vi "18-2.vi"() -> ()   [LabVIEW 2019, in "18.lvlib"]
uses:
  18.lvlib
panel:
  out "Snailfish Number x+y":string
  out "Snailfish Number y":string
  in  "Sample?":bool
  out "Max Snailfish Number Sum Magnitude":u64
  in  "Sample Index":i32
  out "Snailfish Number x":string
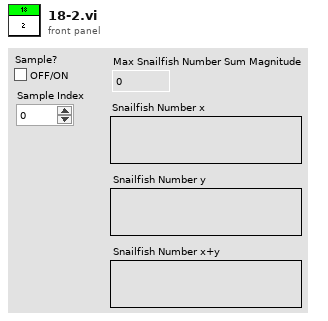
[diagram p1: front panel]
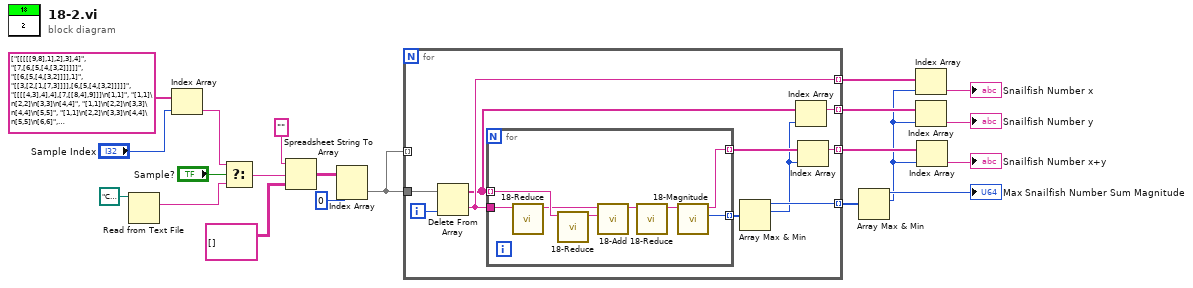
[diagram p0: block diagram]
diagram:
  n1 = Read from Text File(file (use dialog)=path "C:/Users/craig.walker/Documents/GitHub/lv2019-Advent-of-Code-2021/18/input.txt") -> (text=w12:string)  [unwired: 3 in, 3 out]
  n2 = Index Array(array=string[] ["[[[[[9,8],1],2],3],4]", "[7,[6,[5,[4,[3,2]]]]]", "[[6,[5,[4,[3,2]]]],1]", "[[3,[2,[1,[7,3]]]],[6,[5,[4,[3,2]]]]]", "[[[[4,3],4],4],[7,[[8,4],9]]]\n[1,1]", "[1,1]\n[2,2]\n[3,3]\n[4,4]", "[1,1]\n[2,2]\n[3,3]\n[4,4]\n[5,5]", "[1,1]\n[2,2]\n[3,3]\n[4,4]\n[5,5]\n[6,6]", "[[[0,[4,5]],[0,0]],[[[4,5],[2,6]],[9,5]]]\n[7,[[[3,7],[4,3]],[[6,3],[8,8]]]]\n[[2,[[0,8],[3,4]]],[[[6,7],1],[7,[1,6]]]]\n[[[[2,4],7],[6,[0,5]]],[[[6,8],[2,8]],[[2,1],[4,5]]]]\n[7,[5,[[3,8],[1,4]]]]\n[[2,[2,2]],[8,[8,1]]]\n[2,9]\n[1,[[[9,3],9],[[9,0],[0,7]]]]\n[[[5,[7,4]],7],1]\n[[[[4,2],2],6],[8,7]]", "[9,1]", "[[[0,[5,8]],[[1,7],[9,6]]],[[4,[1,2]],[[1,4],2]]]\n[[[5,[2,8]],4],[5,[[9,9],0]]]\n[6,[[[6,2],[5,6]],[[7,6],[4,7]]]]\n[[[6,[0,7]],[0,9]],[4,[9,[9,0]]]]\n[[[7,[6,4]],[3,[1,3]]],[[[5,5],1],9]]\n[[6,[[7,3],[3,2]]],[[[3,8],[5,7]],4]]\n[[[[5,4],[7,7]],8],[[8,3],8]]\n[[9,3],[[9,9],[6,[4,9]]]]\n[[2,[[7,7],7]],[[5,8],[[9,3],[0,2]]]]\n[[[[5,2],5],[8,[3,7]]],[[5,[7,5]],[4,4]]]"], index="Sample Index") -> (element=w13:string)
  n3 = Select(t=w13, s="Sample?", f=w12) -> (s? t:f=w14:string)
  n4 = Spreadsheet String To Array(format string="" ("spreadsheet string"), spreadsheet string=w14, array type (2D Dbl)=string[][] [] ("spreadsheet string")) -> (array=w19:string[][])  [unwired: 1 in]
  n5 = Index Array(array=w19, index (col)=0 ("disabled index (col)")) -> (element=w10:string[])  [unwired: 1 in]
  n6 = for {
    tunnel: w10 -> [w31]
    tunnel: [w25] -> w9 mode=indexing
    tunnel: w10 -> [_] mode=indexing
    tunnel: [w28] -> w7 mode=indexing
    tunnel: [w26] -> w5 mode=indexing
    tunnel: [w23] -> w3 mode=indexing
    i -> [w29]
    n7 = Delete From Array(array=w31, index=w29) -> (deleted portion=w28:string, array with subset deleted=w27:string[])  [unwired: 1 in]
    n8 = for {
      tunnel: w27 -> [w39] mode=indexing
      tunnel: [w35] -> w30 mode=indexing
      tunnel: w28 -> [w38]
      tunnel: [w32] -> w24 mode=indexing
      n9 = call "18-Reduce.vi"("Snailfish Number in"=w38) -> ("Snailfish Number out"=w37:string)  [unwired: 10 in]
      n10 = call "18-Reduce.vi"("Snailfish Number in"=w39) -> ("Snailfish Number out"=w33:string)  [unwired: 10 in]
      n11 = call "18-Add.vi"("Snailfish Number y"=w33, "Snailfish Number x"=w37) -> ("Snailfish Number x+y"=w34:string)  [unwired: 9 in]
      n12 = call "18-Reduce.vi"("Snailfish Number in"=w34) -> ("Snailfish Number out"=w36:string)  [unwired: 10 in]
      n13 = call "18-Magnitude.vi"("Snailfish Number in"=w36) -> ("Snailfish Number Magnitude"=w35:u64, "Snailfish Number out"=w32:string)  [unwired: 9 in]
    }
    n14 = Array Max & Min(array=w30) -> (max value=w25:u64, max index (indices)=w22:i32)  [unwired: 2 out]
    n15 = Index Array(array=w27, index=w22) -> (element=w26:string)
    n16 = Index Array(array=w24, index=w22) -> (element=w23:string)
  }
  n17 = Array Max & Min(array=w9) -> (max value=→"Max Snailfish Number Sum Magnitude":u64, max index (indices)=w2:i32)  [unwired: 2 out]
  n18 = Index Array(array=w7, index=w2) -> (element=→"Snailfish Number x":string)
  n19 = Index Array(array=w5, index=w2) -> (element=→"Snailfish Number y":string)
  n20 = Index Array(array=w3, index=w2) -> (element=→"Snailfish Number x+y":string)
